vi "Choreo_Util_RemoveTrajFileExtension.vi"(11 "FileNameIn":string) -> (3 "FileNameOut":string)   [LabVIEW 2019, in "ChoreoLib.lvlib"]
uses:
  ChoreoLib.lvlib
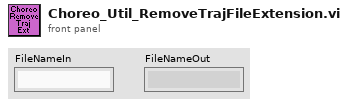
[diagram p1: front panel]
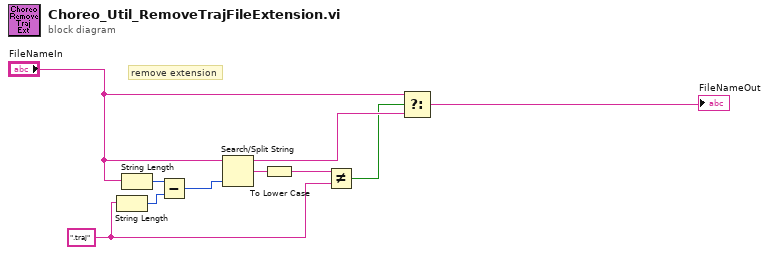
[diagram p0: block diagram]
diagram:
  w7 = ".traj" ("y")
  # "remove extension"
  n1 = String Length(string=w7) -> (length=w6:i32)
  n2 = String Length(string="FileNameIn") -> (length=w1:i32)
  n3 = Subtract(x=w1, y=w6) -> (x-y=w2:i32)
  n4 = Search/Split String(string="FileNameIn", offset (0)=w2) -> (substring before match=w9:string, match + rest of string=w3:string)  [unwired: 1 in, 1 out]
  n5 = To Lower Case(string=w3) -> (all lower case string=w4:string)
  n6 = Not Equal?(x=w4, y=w7) -> (x != y?=w5:bool)
  n7 = Select(t="FileNameIn", s=w5, f=w9) -> (s? t:f=→"FileNameOut":string)
